vi "NXT_HINDBRAIN Beep.vi"(0 "NXT":T1, 1 "Beep Enable":bool, 2 "Tugboat Properties":T2={"_name"="", "_pitch"=0, "_rudderCenter"=0, "_propCenter"=0, "_irServoCenter"=0, "_rudderMin"=1450, "_rudderMax"=1450, "_propMin"=1000, "_propMax"=1000, "_irServoMin"=1000, "_irServoMax"=1000}) -> ()   [LabVIEW 2012, in "Tugboat.lvrbt"]
doc: "Beeps when the 'Beep Enabled' input is set to true at the pitch specified in Tugboat Properties. This is the 'blinky light' for the tugboat."
uses:
  Tugboat.lvrbt
  tugProperties_t.ctl
  <vilib>/NXT/Subs/LVHSConnector.ctl
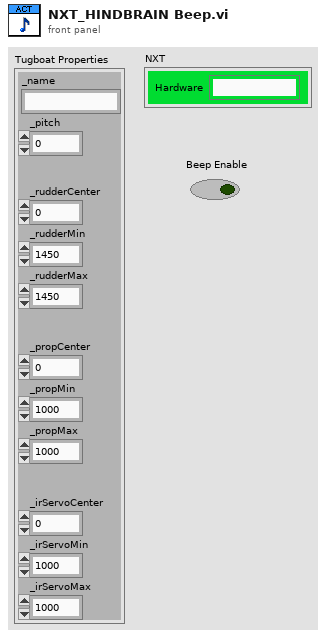
[diagram p1: front panel]
types:
  T1 = typedef "LVHSConnector.ctl" = cluster{"Hardware":string, "Flattened String":string}
  T2 = typedef "tugProperties_t.ctl" = cluster{"_name":string, "_pitch":i32, "_rudderCenter":u16, "_propCenter":u16, "_irServoCenter":u16, "_rudderMin":u16, "_rudderMax":u16, "_propMin":u16, "_propMax":u16, "_irServoMin":u16, "_irServoMax":u16}
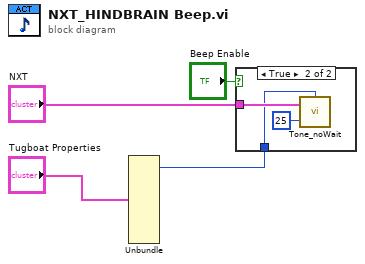
[diagram p0: block diagram]
diagram:
  n1 = Unbundle("Tugboat Properties") -> ("_pitch"=w2:i32)  [unwired: 10 out]
  n2 = case shown="True" "Beep Enable" {
    tunnel: "NXT" -> [_ w7]
    tunnel: w2 -> [_ w6]
    frame False {
    }
    frame True {
      n3 = call <vilib>:"Tone_noWait.vi"("Duration (500 ms)"=u16 25, "NXT"=w7, "Tone (440 Hz)"=w6) -> ()  [unwired: 1 in, 1 out]
    }
  }
